vi "Add Copyright.vi"(0 "File Path":path, 5 "Copyright Text":string="© Company Name", 11 "error in (no error)":errorcluster) -> (15 "error out":errorcluster)   [LabVIEW 2014, in "SLL Add Copyright.lvlib"]
uses:
  SLL Add Copyright.lvlib
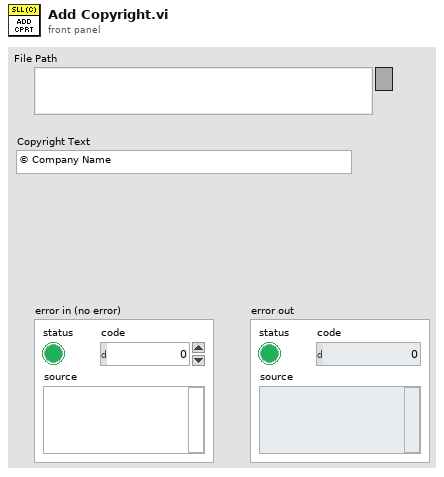
[diagram p1: front panel]
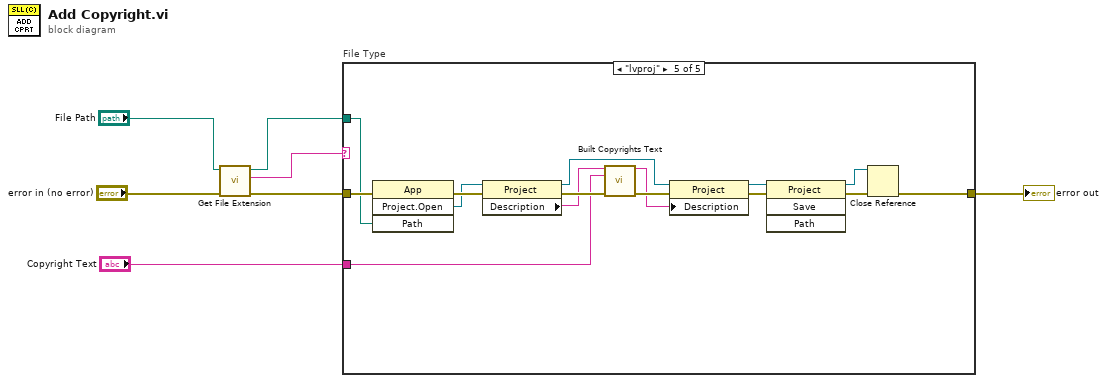
[diagram p0: block diagram]
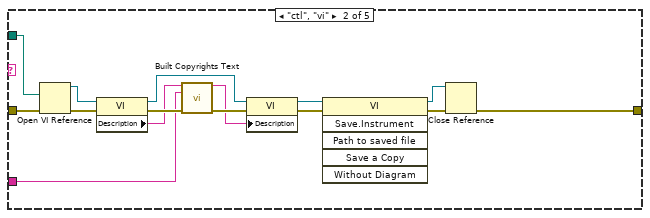
[diagram p3: hidden frame]
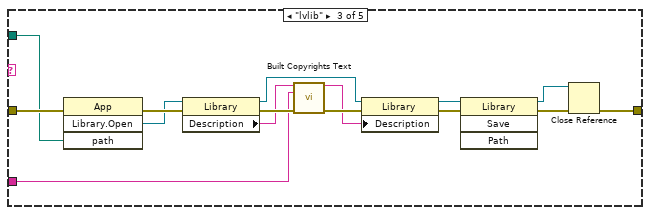
[diagram p4: hidden frame]
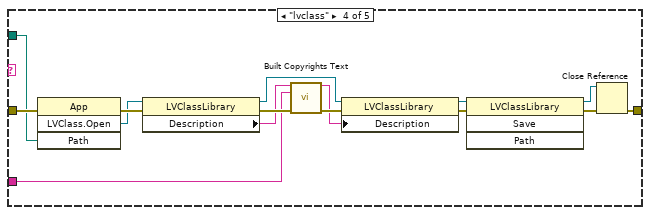
[diagram p5: hidden frame]
diagram:
  n1 = call <vilib>:"Get File Extension.vi"("error in (no error)"="error in (no error)", "file"="File Path") -> ("error out"=w4:errorcluster, "lowercase file extension"=w1:string, "dup file"=w2:path)  [unwired: 5 in, 2 out]
  n2 = case "File Type" shown="\"lvproj\"" w1 {
    tunnel: [w8 w10 w25 w40 w55] -> w6
    tunnel: w4 -> [w8 w23 w38 w53 w68]
    tunnel: w2 -> [_ w21 w36 w51 w66]
    tunnel: "Copyright Text" -> [_ w13 w32 w47 w62]
    frame Default {
    }
    frame "ctl", "vi" {
      n3 = Open VI Reference(vi path=w21, error in (no error)=w23) -> (vi reference=w20:refnum<vi>, error out=w22:errorcluster)  [unwired: 4 in]
      n4 = property class="VI"(reference=w20, error in=w22) -> (reference out=w15:refnum<vi>, error out=w19:errorcluster, "Description"=w17:string)
      n5 = call "Built Copyrights Text.vi"("Description in"=w17, "Licence Text"=w13, "error in"=w19) -> ("Description out"=w14:string, "error out"=w18:errorcluster)  [unwired: 11 in]
      n6 = property class="VI"(reference=w15, error in=w18, "Description"=w14) -> (reference out=w11:refnum<vi>, error out=w16:errorcluster)
      n7 = invoke class="VI" method="Save.Instrument"(reference=w11, error in=w16) -> (reference out=w9:refnum<vi>, error out=w12:errorcluster)  [unwired: 4 in, 4 out]
      n8 = Close Reference(reference=w9, error in (no error)=w12) -> (error out=w10:errorcluster)
    }
    frame "lvlib" {
      n9 = invoke class="App" method="Library.Open"(error in=w38, "path"=w36) -> (error out=w37:errorcluster, "Open Library"=w35:refnum<vi>)  [unwired: 2 in, 2 out]
      n10 = property class="Library"(reference=w35, error in=w37) -> (reference out=w28:refnum<vi>, error out=w34:errorcluster, "Description"=w33:string)
      n11 = call "Built Copyrights Text.vi"("Description in"=w33, "Licence Text"=w32, "error in"=w34) -> ("Description out"=w29:string, "error out"=w31:errorcluster)  [unwired: 11 in]
      n12 = property class="Library"(reference=w28, error in=w31, "Description"=w29) -> (reference out=w26:refnum<vi>, error out=w30:errorcluster)
      n13 = invoke class="Library" method="Save"(reference=w26, error in=w30) -> (reference out=w24:refnum<vi>, error out=w27:errorcluster)  [unwired: 2 in, 2 out]
      n14 = Close Reference(reference=w24, error in (no error)=w27) -> (error out=w25:errorcluster)
    }
    frame "lvclass" {
      n15 = invoke class="App" method="LVClass.Open"(error in=w53, "Path"=w51) -> (error out=w52:errorcluster, "LVClass.Open"=w50:refnum<vi>)  [unwired: 2 in, 2 out]
      n16 = property class="LVClassLibrary"(reference=w50, error in=w52) -> (reference out=w43:refnum<vi>, error out=w49:errorcluster, "Description"=w48:string)
      n17 = call "Built Copyrights Text.vi"("Description in"=w48, "Licence Text"=w47, "error in"=w49) -> ("Description out"=w44:string, "error out"=w46:errorcluster)  [unwired: 11 in]
      n18 = property class="LVClassLibrary"(reference=w43, error in=w46, "Description"=w44) -> (reference out=w41:refnum<vi>, error out=w45:errorcluster)
      n19 = invoke class="LVClassLibrary" method="Save"(reference=w41, error in=w45) -> (reference out=w39:refnum<vi>, error out=w42:errorcluster)  [unwired: 2 in, 2 out]
      n20 = Close Reference(reference=w39, error in (no error)=w42) -> (error out=w40:errorcluster)
    }
    frame "lvproj" {
      n21 = invoke class="App" method="Project.Open"(error in=w68, "Path"=w66) -> (error out=w67:errorcluster, "Project:Open"=w65:refnum<vi>)  [unwired: 2 in, 2 out]
      n22 = property class="Project"(reference=w65, error in=w67) -> (reference out=w58:refnum<vi>, error out=w64:errorcluster, "Description"=w63:string)
      n23 = call "Built Copyrights Text.vi"("Description in"=w63, "Licence Text"=w62, "error in"=w64) -> ("Description out"=w59:string, "error out"=w61:errorcluster)  [unwired: 11 in]
      n24 = property class="Project"(reference=w58, error in=w61, "Description"=w59) -> (reference out=w56:refnum<vi>, error out=w60:errorcluster)
      n25 = invoke class="Project" method="Save"(reference=w56, error in=w60) -> (reference out=w54:refnum<vi>, error out=w57:errorcluster)  [unwired: 2 in, 2 out]
      n26 = Close Reference(reference=w54, error in (no error)=w57) -> (error out=w55:errorcluster)
    }
  }
  "error out" <- w6
